vi "Write to Hardware.vi"(7 "Valid Triggers":bool, 8 "error in (no error)":errorcluster, 9 "Trigger Values":dbl[](array[numeric]), 10 "Values in":dbl[](array[numeric]), 11 "Monitor Execution Unit Implementation in":refnum<class "Monitor Execution Unit.lvclass">) -> (0 "error out":errorcluster, 1 "Trigger Values out":dbl[](array[numeric]), 2 "Values out":dbl[](array[numeric]), 3 "Monitor Execution Unit Implementation out":refnum<class "Monitor Execution Unit.lvclass">)   [LabVIEW 2020, in "AIM ARINC 664 Engine.lvlib" / "Implementation.lvlib" / "Monitor Execution Unit.lvclass"]
uses:
  Monitor Execution Unit.lvclass
  Logging/Frame Logging/Frame Logging.lvlib
  <vilib>/Utility/SystemLogging/NI_SystemLogging.lvlib
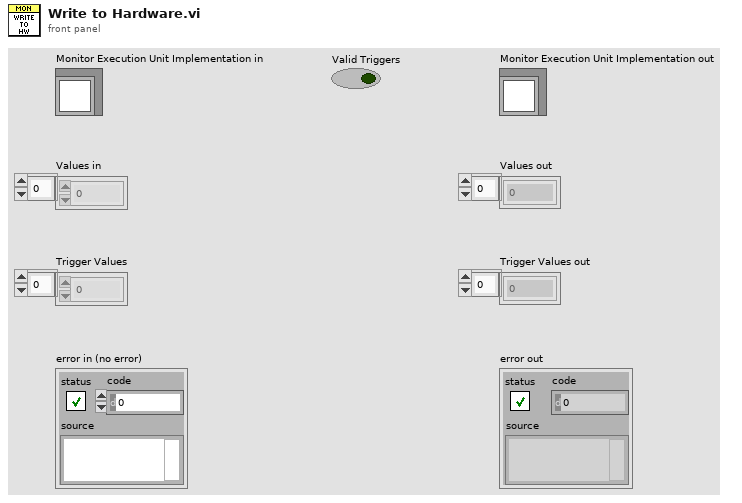
[diagram p1: front panel]
types:
  T1 = typedef "Frame Logging.lvlib/Log_Producer.ctl" = cluster{"Configured":bool, "message queue in":refnum<queue>, "StopNotification":refnum<notifier>}
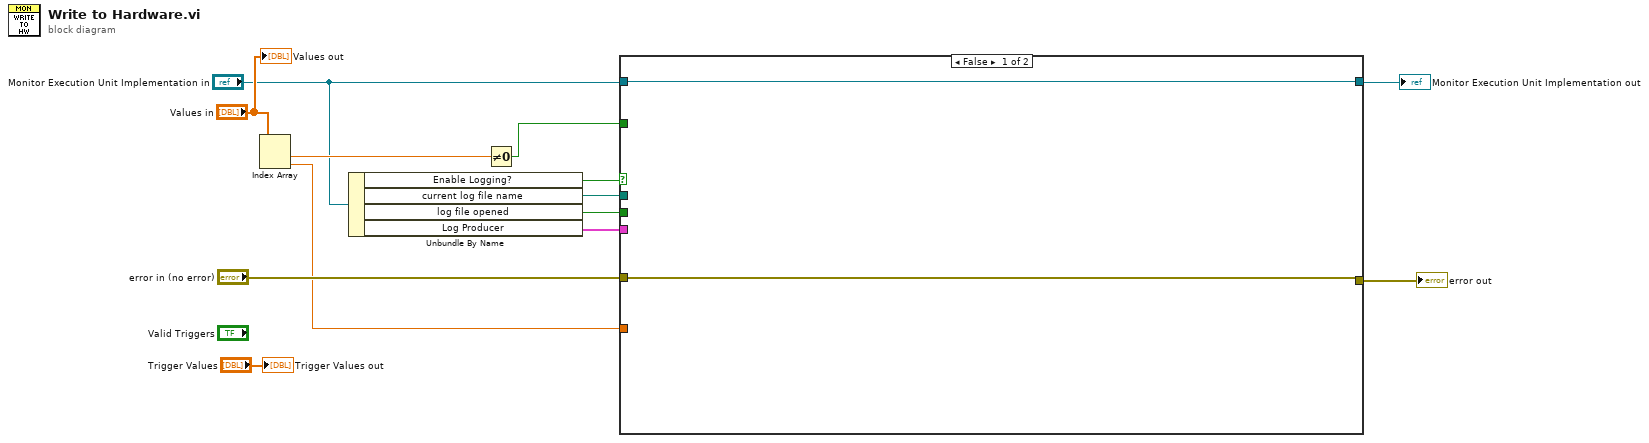
[diagram p0: block diagram]
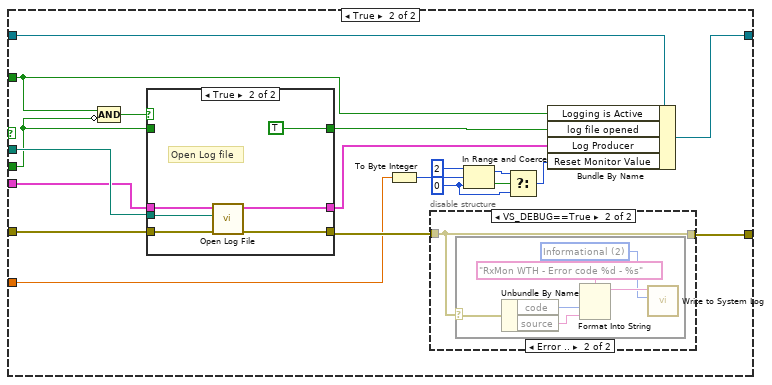
[diagram p2: hidden frame]
diagram:
  n1 = Index Array(array="Values in") -> (element #1=w10:dbl, element #2=w2:dbl)  [unwired: 2 in]
  n2 = Unbundle By Name("Monitor Execution Unit Implementation in") -> ("Enable Logging?"=w1:bool, "current log file name"=w7:path, "log file opened"=w5:bool, "Log Producer"=w4:T1)
  n3 = Not Equal To 0?(x=w10) -> (x != 0?=w8:bool)
  n4 = case shown="False" w1 {
    tunnel: [w15 w34] -> w12
    tunnel: "Monitor Execution Unit Implementation in" -> [w15 w32]
    tunnel: w8 -> [_ w31]
    tunnel: w7 -> [_ w30]
    tunnel: "error in (no error)" -> [w14 w29]
    tunnel: w5 -> [_ w27]
    tunnel: w4 -> [_ w26]
    tunnel: [w14 w23] -> w3
    tunnel: w2 -> [_ w22]
    frame False {
    }
    frame True {
      w16 = i8 0 ("lower limit")
      n5 = Compound Arithmetic op=AND(w31, invert w27) -> (w33:bool)
      n6 = case shown="True" w33 {
        tunnel: [w44 TRUE] -> w28
        tunnel: w30 -> [_ w48]
        tunnel: w29 -> [w45 w49]
        tunnel: [w45 w47] -> w24
        tunnel: w27 -> [w44 _]
        tunnel: w26 -> [w43 w50]
        tunnel: [w43 w46] -> w25
        frame False {
        }
        frame True {
          # "Open Log file"
          n7 = call "Open Log File.vi"("error in"=w49, "File Path"=w48, "Log Producer in"=w50) -> ("error out"=w47:errorcluster, "Log Producer out"=w46:T1)  [unwired: 7 in]
        }
      }
      n8 = To Byte Integer(number=w22) -> (8bit integer=w21:i8)
      n9 = disable-structure shown="VS_DEBUG==True" {
        disable-tunnel: w24 -> [w35 w36]
        disable-tunnel: [w35 w36] -> w23
        frame condition #0 (active) {
        }
        frame condition #1 {
          n10 = case shown="Error .." w36 {
            selector: w36 -> [_ w37]
            frame No Error {
            }
            frame Error {
              w40 = 2 items=["Error", "Warning", "Informational"] ("severity")
              n11 = Unbundle By Name(w37) -> ("code"=w39:i32, "source"=w38:string)
              n12 = Format Into String(format string="RxMon WTH - Error code %d - %s", w39, w38) -> (resulting string=w41:string)  [unwired: 2 in, 1 out]
              n13 = call <vilib>:"Write to System Log.vi"("severity"=w40, "message"=w41) -> ()  [unwired: 9 in, 1 out]
            }
          }
        }
      }
      n14 = In Range and Coerce(upper limit=i8 2, x=w21, lower limit=w16) -> (coerced(x)=w18:i8, In Range?=w19:bool)
      n15 = Select(t=w18, s=w19, f=w16) -> (s? t:f=w17:i8)
      n16 = Bundle By Name(cluster=w32, "Logging is Active"=w31, "log file opened"=w28, "Log Producer"=w25, "Reset Monitor Value"=w17) -> (w34:refnum<class "Monitor Execution Unit.lvclass">)
    }
  }
  "error out" <- w3
  "Monitor Execution Unit Implementation out" <- w12
  "Values out" <- "Values in"
  "Trigger Values out" <- "Trigger Values"
